vi "Delete_unwanted_rows.vi"(1 "Selected Rows":i32[](array[numeric]), 2 "Filename":path) -> ()   [LabVIEW 2020]
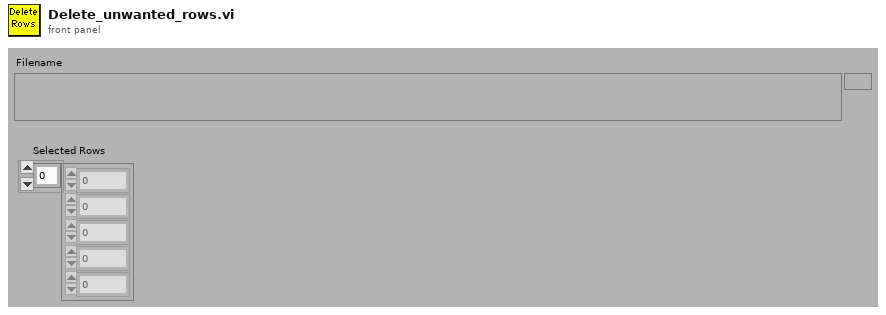
[diagram p1: front panel]
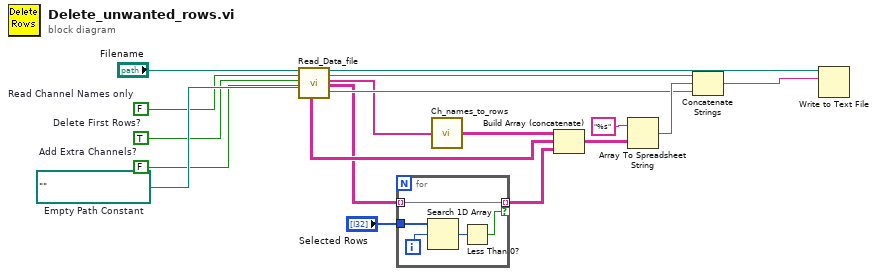
[diagram p0: block diagram]
diagram:
  w2 = TRUE  # Delete First Rows?
  w6 = FALSE  # Add Extra Channels?
  w16 = FALSE  # Read Channel Names only
  w17 = path ""  # Empty Path Constant
  n1 = call "Read_Data_file.vi"("Results file"="Filename", "Read Channel Names only"=w16, "Delete First Rows?"=w2, "Add Extra Channels?"=w6, "Template File"=w17) -> ("Deleted Rows"=w7:string[][], "Results file Out"=w8:path, "String Before"=w14:string, "Ch names Out"=w1:string[], "Channel Values Out"=w4:string[][], "String After"=w10:string)  [unwired: 2 in, 7 out]
  n2 = for {
    tunnel: "Selected Rows" -> [w23]
    tunnel: w4 -> [w20] mode=indexing
    tunnel: [w20] -> w3 mode=indexing if=w19
    i -> [w22]
    n3 = Search 1D Array(1D array=w23, element=w22) -> (index of element=w21:i32)  [unwired: 1 in]
    n4 = Less Than 0?(x=w21) -> (x < 0?=w19:bool)
  }
  n5 = call "Ch_names_to_rows.vi"("Channel Names"=w1) -> ("3 Row names"=w13:string[][])
  n6 = Build Array (concatenate)(w13, w7, w3) -> (w12:string[][])
  n7 = Array To Spreadsheet String(array=w12, 3:"%s" ("format string")) -> (spreadsheet string=w11:string)  [unwired: 1 in]
  n8 = Concatenate Strings(w14, w11, w10) -> (w9:string)
  n9 = Write to Text File(file (use dialog)=w8, text=w9) -> ()  [unwired: 2 in, 3 out]
